vi "Mux I16xN.vi"(0 "i16xn in":fxp<+/-,18,1>[](array[numeric]), 5 "index":i32, 9 "input valid":bool[](array[boolean])) -> (4 "i16 out":fxp<+/-,18,1> format="%.18g", 10 "output valid":bool)   [LabVIEW 2017, in "Lock-In Amplifier Example FPGA.lvlib"]
uses:
  Lock-In Amplifier Example FPGA.lvlib
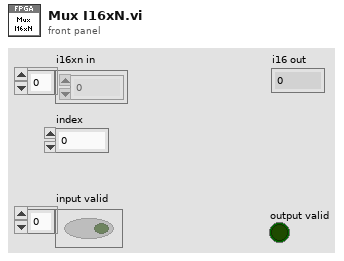
[diagram p1: front panel]
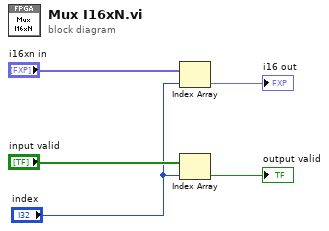
[diagram p0: block diagram]
diagram:
  n1 = Index Array(array="i16xn in", index="index") -> (element=→"i16 out":fxp<+/-,18,1>)
  n2 = Index Array(array="input valid", index="index") -> (element=→"output valid":bool)
